vi "usun_zera.vi"(11 "Tablica współczynników":dbl[](array[numeric])) -> (0 "ilość zer":i32, 3 "Współczynniki":dbl[](array[numeric]))   [LabVIEW 2020]
doc: "usuwa zerowe współczynniki"
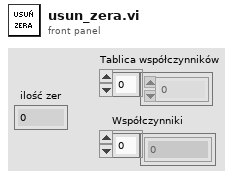
[diagram p1: front panel]
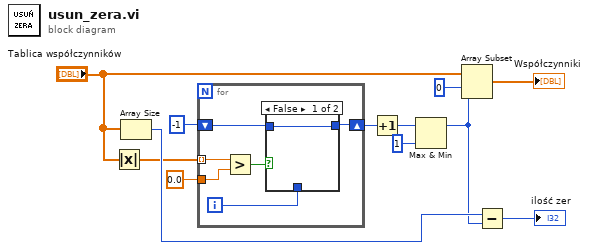
[diagram p0: block diagram]
diagram:
  n1 = Absolute Value(x="Tablica współczynników") -> (abs(x)=w9:dbl[])
  n2 = Array Size(array="Tablica współczynników") -> (size(s)=w11:i32)
  n3 = for {
    shift-right: [w17] -> w7
    shift-left: -1 -> [w16]
    tunnel: w9 -> [w14] mode=indexing
    tunnel: 0.0 ("threshold") -> [w13]
    i -> [w18]
    n4 = Greater?(x=w14, y=w13) -> (0:w15:bool)
    n5 = case shown="False" w15 {
      tunnel: w18 -> [_ w20]
      tunnel: [w19 w20] -> w17
      tunnel: w16 -> [w19 _]
      frame False {
      }
      frame True {
      }
    }
  }
  n6 = Increment(x=w7) -> (x+1=w5:i32)
  n7 = Max & Min(x=w5, y=1) -> (max(x,y)=w3:i32)  [unwired: 1 out]
  n8 = Array Subset(array="Tablica współczynników", index=0, length=w3) -> (→"Współczynniki":dbl[])
  n9 = Subtract(x=w11, y=w3) -> (x-y=→"ilość zer":i32)
